vi "Harvest_RD_Filenames.vi"() -> ()   [LabVIEW 2010]
uses:
  Controls/File_Selector_Type.ctl
panel:
  in  "Output File":path
  out "Checking":i32
  out "Choosen path":path
  in  "Previous Choice":path
  in  "File Type":string
  in  "At Dialog Prompt Post Process":T1
  in  "Search String":string
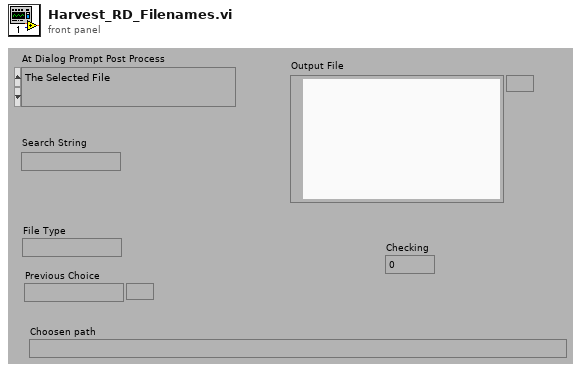
[diagram p1: front panel]
types:
  T1 = typedef "File_Selector_Type.ctl" = enum16{"The Selected File", "The Selected Folder", "Files containing the search string in the selected folder", "All files listed in selected file"}
  T2 = enum32{"existing file", "new file", "new or existing file", "existing dir", "new dir", "new or existing dir", "existing file (use LLBs)", "new file (use LLBs)", "new or existing file (use LLBs)", "new or existing file or directory (use LLBs)"}
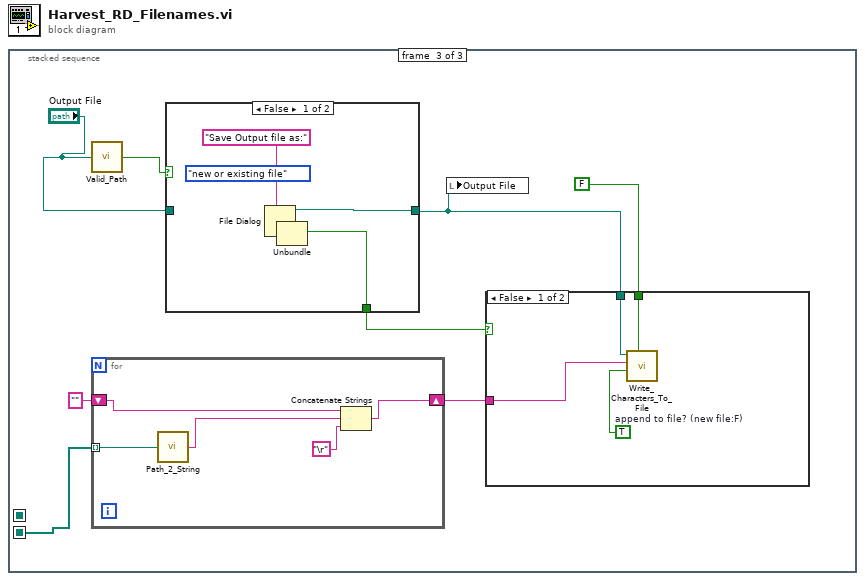
[diagram p0: block diagram]
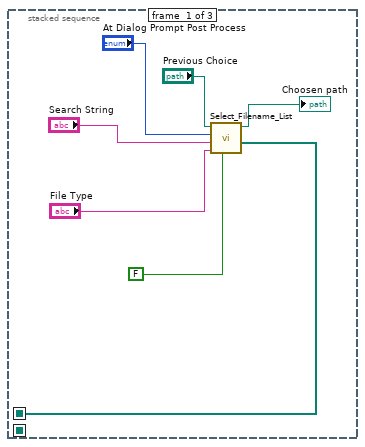
[diagram p2: hidden frame]
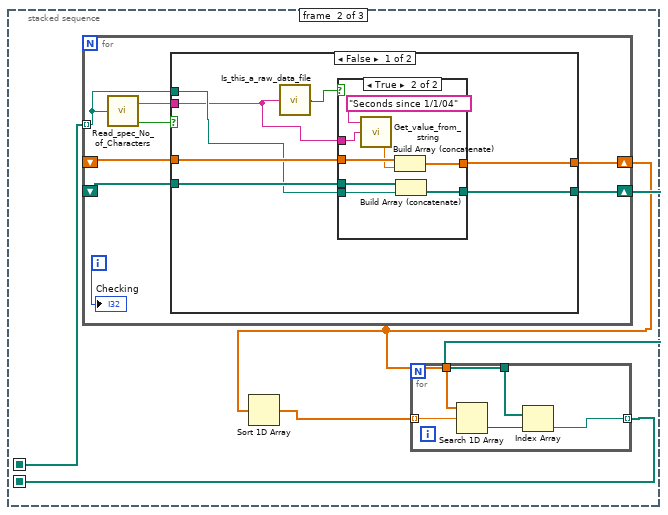
[diagram p3: hidden frame]
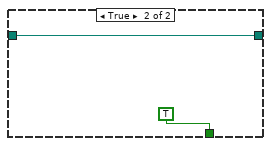
[diagram p7: hidden frame]
diagram:
  n1 = stacked-sequence {
    seq-local: [w1 _ _] -> [_ w11 _]
    seq-local: [_ w8 _] -> [_ _ w52]
    frame #0 {
      n2 = call "Select_Filename_List.vi"("No dialogs"=FALSE, "File Type"="File Type", "Search String"="Search String", "At Dialog Prompt Post Process"="At Dialog Prompt Post Process", "Previous Choice"="Previous Choice") -> ("Selected files"=w1:path[], "Choosen path"=→"Choosen path":path)  [unwired: 1 in, 1 out]
    }
    frame #1 {
      n3 = for {
        tunnel: w11 -> [w20] mode=indexing
        shift-right: [w24] -> w9
        shift-left: _ -> [w25]
        shift-right: [w22] -> w10
        shift-left: _ -> [w23]
        i -> [w21]
        n4 = call "Read_spec_No_of_Characters.vi"("Filename"=w20) -> ("character string"=w19:string, "Error?"=w18:bool)
        n5 = case shown="False" w18 {
          tunnel: w25 -> [w32 w44]
          tunnel: [w31 w44] -> w24
          tunnel: w23 -> [w30 w43]
          tunnel: [w29 w43] -> w22
          tunnel: w20 -> [w27 _]
          tunnel: w19 -> [w26 _]
          frame False {
            n6 = call "Is_this_a_raw_data_file.vi"("character string"=w26) -> ("Raw Dat File?"=w28:bool)  [unwired: 2 in]
            n7 = case shown="True" w28 {
              tunnel: w32 -> [w34 w40]
              tunnel: [w34 w42] -> w31
              tunnel: w30 -> [w33 w38]
              tunnel: w27 -> [_ w37]
              tunnel: [w33 w36] -> w29
              tunnel: w26 -> [_ w35]
              frame False {
              }
              frame True {
                n8 = call "Get_value_from_string.vi"("Input string"=w35, "Variable name"="Seconds since 1/1/04") -> ("Value"=w39:dbl)  [unwired: 1 in, 1 out]
                n9 = Build Array (concatenate)(w40, w39) -> (w42:dbl[])
                n10 = Build Array (concatenate)(w38, w37) -> (w36:path[])
              }
            }
          }
          frame True {
          }
        }
        "Checking" <- w21
      }
      n11 = Sort 1D Array(array=w9) -> (sorted array=w12:dbl[])
      n12 = for {
        tunnel: w9 -> [w17]
        tunnel: w12 -> [w16] mode=indexing
        tunnel: w10 -> [w15]
        tunnel: [w14] -> w8 mode=indexing
        n13 = Search 1D Array(1D array=w17, element=w16) -> (index of element=w13:i32)  [unwired: 1 in]
        n14 = Index Array(array=w15, index=w13) -> (element=w14:path)
      }
    }
    frame #2 {
      n15 = call "Valid_Path.vi"("Filename"="Output File") -> ("Valid Path?"=w48:bool)
      n16 = for {
        tunnel: w52 -> [w67] mode=indexing
        shift-right: [w65] -> w50
        shift-left: "" -> [w66]
        n17 = call "Path_2_String.vi"("Real Path"=w67) -> ("Path String"=w64:string)
        n18 = Concatenate Strings(w66, w64, "\r") -> (w65:string)
      }
      n19 = case shown="False" w48 {
        tunnel: [w59 w62] -> w45
        tunnel: "Output File" -> [_ w62]
        tunnel: [w58 TRUE ("cancelled")] -> w46
        frame False {
          (unwired) T2."new or existing file" ("select mode (2)")
          n20 = File Dialog(7:"Save Output file as:" ("prompt")) -> (0:w57:errorcluster, 1:w58:bool, 3:w59:path)  [unwired: 6 in, 1 out]
          n21 = Unbundle(w57) -> ()  [unwired: 3 out]
        }
        frame True {
        }
      }
      n22 = local write "Output File"(w45) -> ()
      n23 = case shown="False" w46 {
        tunnel: w50 -> [w56 _]
        tunnel: FALSE ("advisory dialog? (display:T)") -> [w55 _]
        tunnel: w45 -> [w53 _]
        frame False {
          w54 = TRUE  # append to file? (new file:F)
          n24 = call "Write_Characters_To_File.vi"("file path (dialog if empty)"=w53, "advisory dialog? (display:T)"=w55, "character string"=w56, "append to file? (new file:F)"=w54) -> ()  [unwired: 4 in, 1 out]
        }
        frame True {
        }
      }
    }
  }
